vi "numCmd_Send_Chassis.vi"(7 "Command Name":string, 11 "Chassis Speeds":T1 {"vOmega" format="%10.3f"; "vY" format="%10.3f"; "vX" format="%10.3f"}) -> (0 "error out":errorcluster)   [LabVIEW 2019, in "Trajectory_Library.lvlib"]
uses:
  Trajectory_Library.lvlib
  TypeDef/CHASSIS_SPEEDS.ctl
  numCmd_ObtainQueue_Generic.vi
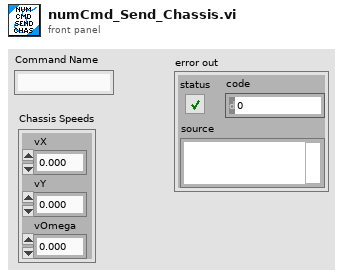
[diagram p1: front panel]
types:
  T1 = typedef "Trajectory_Library.lvlib/CHASSIS_SPEEDS.ctl" = cluster{"vX":dbl, "vY":dbl, "vOmega":dbl}
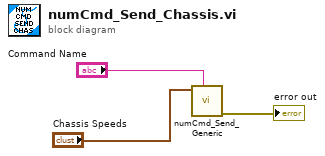
[diagram p0: block diagram]
diagram:
  n1 = call "numCmd_Send_Generic.vi"("Command Name"="Command Name", "Value"="Chassis Speeds") -> ("error out"=→"error out":errorcluster)  [unwired: 9 in]
